vi "Initialize.vi"(8 "error in (no error)":errorcluster, 9 "Reset (True)":bool=TRUE, 10 "ID Query (True)":bool=TRUE, 11 "VISA resource name":refnum<visa-resource-name>) -> (0 "error out":errorcluster, 3 "VISA resource name out":refnum<visa-resource-name>)   [LabVIEW 2017, in "ADCMT7351_ADC.lvlib"]
doc: "Establishes communication with the instrument and optionally performs an instrument identification query and/or an instrument reset. It also places the instrument in a default state needed for other instrument driver operations. Therefore, call this VI before calling other instrument driver VIs for this instrument. Generally, you need to call the <B>Initialize VI</B> only once at the beginning of an application."
uses:
  ADCMT7351_ADC.lvlib
  <vilib>/regexp/Match Regular Expression.xnode
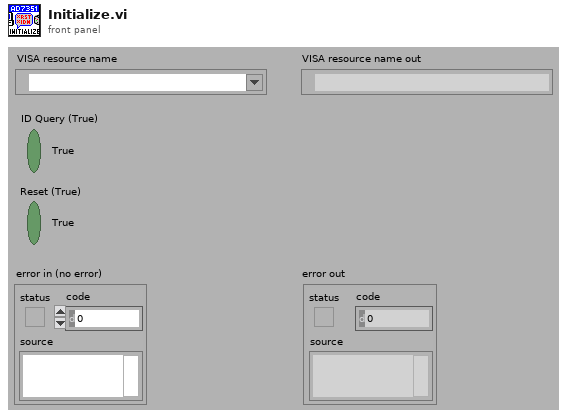
[diagram p1: front panel]
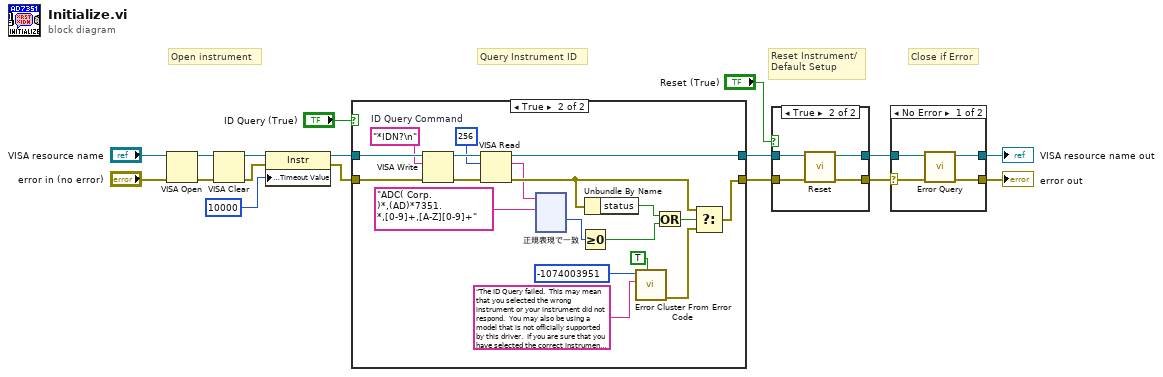
[diagram p0: block diagram]
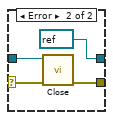
[diagram p2: hidden frame]
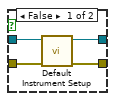
[diagram p3: hidden frame]
diagram:
  # "Close if Error"
  # "Query Instrument ID"
  # "Reset Instrument/\nDefault Setup"
  # "Open instrument"
  n1 = VISA Open(error in (no error)="error in (no error)", VISA resource name="VISA resource name") -> (VISA resource name=w10:refnum<visa-resource-name>, error out=w9:errorcluster)  [unwired: 3 in]
  n2 = VISA Clear(VISA resource name=w10, error in (no error)=w9) -> (VISA resource name out=w8:refnum<visa-resource-name>, error out=w7:errorcluster)
  n3 = property class="Instr"(reference=w8, error in=w7, "General Settings:Timeout Value"=u32 10000) -> (reference out=w5:refnum<visa-resource-name>, error out=w4:errorcluster)
  n4 = case shown="True" "ID Query (True)" {
    tunnel: [w18 w38] -> w16
    tunnel: [w19 w35] -> w17
    tunnel: w5 -> [w19 w36]
    tunnel: w4 -> [w18 w37]
    frame False {
    }
    frame True {
      w22 = "*IDN?\n"  # ID Query Command
      n5 = VISA Write(VISA resource name=w36, write buffer=w22, error in (no error)=w37) -> (VISA resource name out=w34:refnum<visa-resource-name>, error out=w33:errorcluster)  [unwired: 1 out]
      n6 = VISA Read(VISA resource name=w34, byte count=u32 256, error in (no error)=w33) -> (VISA resource name out=w35:refnum<visa-resource-name>, read buffer=w20:string, error out=w27:errorcluster)  [unwired: 1 out]
      n7 = xnode "正規表現で一致"("input string"=w20, "regular expression"="ADC( Corp.)*,(AD)*7351.*,[0-9]+,[A-Z][0-9]+") -> ("offset past match"=w23:i32)  [unwired: 4 in, 4 out]
      n8 = Greater Or Equal To 0?(x=w23) -> (x >= 0?=w25:bool)
      n9 = Unbundle By Name(w27) -> ("status"=w26:bool)
      n10 = call <vilib>:"Error Cluster From Error Code.vi"("show call chain? (False)"=TRUE, "error message (\"\")"="The ID Query failed.  This may mean that you selected the wrong instrument or your instrument did not respond.  You may also be using a model that is not officially supported by this driver.  If you are sure that you have selected the correct instrument and it is responding, try disabling the ID Query." ("Source (VI Name)"), "error code (0)"=-1074003951 ("Code")) -> ("error out"=w31:errorcluster)  [unwired: 6 in]
      n11 = Or(x=w26, y=w25) -> (x .or. y?=w24:bool)
      n12 = Select(t=w27, s=w24, f=w31) -> (s? t:f=w38:errorcluster)
    }
  }
  n13 = case shown="True" "Reset (True)" {
    tunnel: w16 -> [w155 w157]
    tunnel: [w154 w160] -> w2
    tunnel: w17 -> [w156 w158]
    tunnel: [w153 w159] -> w3
    frame False {
      n14 = call "Default Instrument Setup.vi"("error in (no error)"=w155, "VISA resource name"=w156) -> ("error out"=w154:errorcluster, "VISA resource name out"=w153:refnum<visa-resource-name>)  [unwired: 8 in]
    }
    frame True {
      n15 = call "Reset.vi"("error in (no error)"=w157, "VISA resource name"=w158) -> ("error out"=w160:errorcluster, "VISA resource name out"=w159:refnum<visa-resource-name>)  [unwired: 8 in]
    }
  }
  n16 = case shown="No Error" w2 {
    selector: w2 -> [w162 w166]
    tunnel: w3 -> [w161 w167]
    tunnel: [w164 refnum<visa-resource-name> refnum ("VISA resource name out")] -> w6
    tunnel: [w163 w168] -> w1
    frame No Error {
      n17 = call "Error Query.vi"("error in (no error)"=w162, "VISA resource name"=w161) -> ("error out"=w163:errorcluster, "VISA resource name out"=w164:refnum<visa-resource-name>)  [unwired: 6 in, 2 out]
    }
    frame Error {
      n18 = call "Close.vi"("error in (no error)"=w166, "VISA resource name"=w167) -> ("error out"=w168:errorcluster)  [unwired: 9 in]
    }
  }
  "VISA resource name out" <- w6
  "error out" <- w1
